vi "Motor-Check.vi"(8 "error in (no error)":errorcluster, 11 "Automation Refnum in":refnum<k7>) -> (0 "error out":errorcluster, 3 "Automation Refnum out":refnum<k7>)   [LabVIEW 2021]
doc: "André Romero - 2019\nandretec@ifsc.usp.br\nIFSC - USP"
panel:
  out "Identify":i32
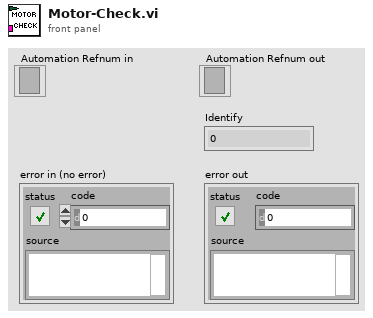
[diagram p1: front panel]
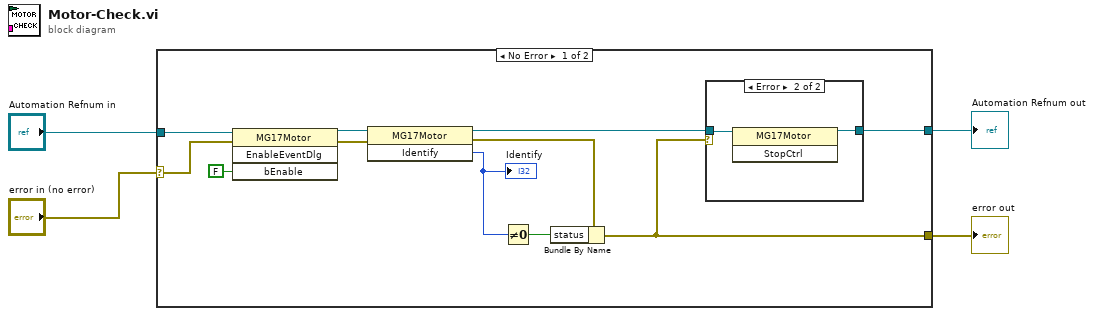
[diagram p0: block diagram]
diagram:
  n1 = case shown="No Error" "error in (no error)" {
    selector: "error in (no error)" -> [w5 w19]
    tunnel: "Automation Refnum in" -> [w11 w20]
    tunnel: [w9 w20] -> w3
    tunnel: [w7 w19] -> w2
    frame No Error {
      n2 = invoke class="MG17Motor" method="EnableEventDlg"(reference=w11, error in=w5, "bEnable"=FALSE) -> (reference out=w13:refnum<k7>, error out=w6:errorcluster)  [unwired: 1 in, 2 out]
      n3 = invoke class="MG17Motor" method="Identify"(reference=w13, error in=w6) -> (reference out=w10:refnum<k7>, error out=w8:errorcluster, "Identify"=w14:i32)  [unwired: 1 in]
      "Identify" <- w14
      n4 = Not Equal To 0?(x=w14) -> (x != 0?=w15:bool)
      n5 = Bundle By Name(cluster=w8, "status"=w15) -> (w7:errorcluster)
      n6 = case shown="Error" w7 {
        tunnel: w10 -> [w16 w18]
        tunnel: [w16 w17] -> w9
        frame No Error {
        }
        frame Error {
          n7 = invoke class="MG17Motor" method="StopCtrl"(reference=w18) -> (reference out=w17:refnum<k7>)  [unwired: 2 in, 2 out]
        }
      }
    }
    frame Error {
    }
  }
  "error out" <- w2
  "Automation Refnum out" <- w3
